vi "addBroadcastFreezeSensorValuesFrame.vi"(0 "FAILC in":refnum<class "FAILC.lvclass">, 5 "ModbusBuffer in":refnum<class "ModbusBuffer.lvclass">, 7 "Subnet":u8, 9 "BroadcastCounter":u8, 11 "error in (no error)":errorcluster) -> (4 "FAILC out":refnum<class "FAILC.lvclass">, 6 "ModbusBuffer out":refnum<class "ModbusBuffer.lvclass">, 15 "error out":errorcluster)   [LabVIEW 2016, in "RTFAILC.lvlib" / "FAILC.lvclass"]
uses:
  FAILC.lvclass
  Common_RT_Modbus/ModbusBuffer/ModbusBuffer.lvclass
  FAILC.lvclass/FAILC.ctl
  Common_RT_Modbus/ModbusBuffer/ModbusBuffer.lvclass/ModbusBuffer.ctl
  Common_RT_Modbus/ModbusBuffer/writeByteInstruction.vi
  Common_RT_Modbus/ModbusBuffer/calculateCRC.vi
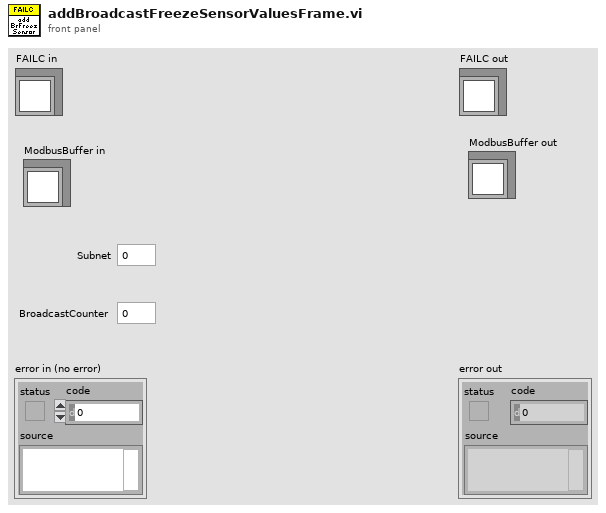
[diagram p1: front panel]
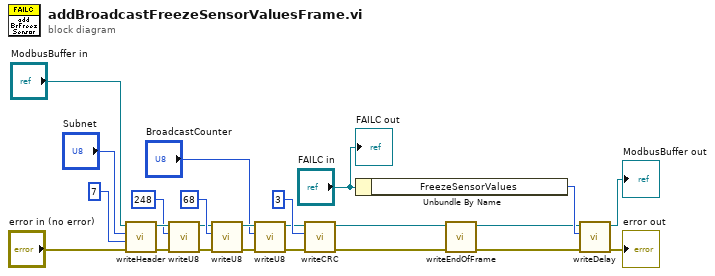
[diagram p0: block diagram]
diagram:
  n1 = call "writeHeader.vi"("error in (no error)"="error in (no error)", "Length"=u16 7, "Subnet"="Subnet", "ModbusBuffer in"="ModbusBuffer in") -> ("error out"=w20:errorcluster, "ModbusBuffer out"=w23:refnum<class "ModbusBuffer.lvclass">)  [unwired: 6 in]
  n2 = call "writeU8.vi"("error in (no error)"=w20, "Input"=u8 248, "ModbusBuffer in"=w23) -> ("error out"=w19:errorcluster, "ModbusBuffer out"=w9:refnum<class "ModbusBuffer.lvclass">)  [unwired: 7 in]
  n3 = call "writeU8.vi"("error in (no error)"=w19, "Input"=u8 68 ("Function"), "ModbusBuffer in"=w9) -> ("error out"=w14:errorcluster, "ModbusBuffer out"=w13:refnum<class "ModbusBuffer.lvclass">)  [unwired: 7 in]
  n4 = call "writeU8.vi"("error in (no error)"=w14, "Input"="BroadcastCounter", "ModbusBuffer in"=w13) -> ("error out"=w10:errorcluster, "ModbusBuffer out"=w11:refnum<class "ModbusBuffer.lvclass">)  [unwired: 7 in]
  n5 = call "writeCRC.vi"("error in (no error)"=w10, "Length"=3, "ModbusBuffer in"=w11) -> ("error out"=w18:errorcluster, "ModbusBuffer out"=w22:refnum<class "ModbusBuffer.lvclass">)  [unwired: 7 in]
  n6 = Unbundle By Name("FAILC in") -> ("FreezeSensorValues"=w8:u32)
  n7 = call "writeEndOfFrame.vi"("error in (no error)"=w18, "ModbusBuffer in"=w22) -> ("error out"=w6:errorcluster, "ModbusBuffer out"=w7:refnum<class "ModbusBuffer.lvclass">)  [unwired: 8 in]
  n8 = call "writeDelay.vi"("error in (no error)"=w6, "Delay(us)"=w8, "ModbusBuffer in"=w7) -> ("error out"=→"error out":errorcluster, "ModbusBuffer out"=→"ModbusBuffer out":refnum<class "ModbusBuffer.lvclass">)  [unwired: 7 in]
  "FAILC out" <- "FAILC in"
